vi "Compare Topologies.vi"(8 "error in (no error)":errorcluster, 9 "Modified Base Topology":path, 11 "Base Topology":path) -> (0 "error out":errorcluster, 3 "Differences":T2(array[cluster]) {"path capability" items=["Path Available"=1, "Path Exists"=2, "Path Unsupported"=3, "Resource in Use"=4, "Source Conflict"=5, "Channel Not Available"=6]; "path capability" items=["Path Available"=1, "Path Exists"=2, "Path Unsupported"=3, "Resource in Use"=4, "Source Conflict"=5, "Channel Not Available"=6]})   [LabVIEW 2017]
uses:
  <vilib>/SLSC_Switch/Path Capability.ctl
  <vilib>/SLSC_Switch/SLSC Switch.lvlib
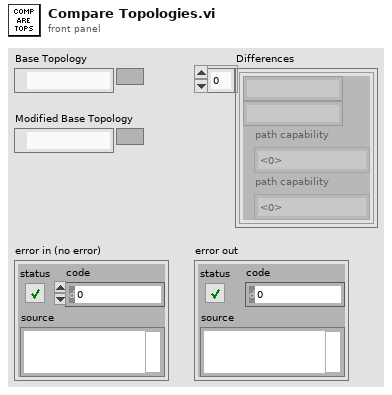
[diagram p1: front panel]
types:
  T1 = typedef "SLSC Switch.lvlib/Path Capability.ctl" = i32
  T2 = cluster{string, string, "path capability":T1, "path capability":T1}[]
  T3 = typedef "nislscslSession.ctl" = refnum<k20>
  T4 = cluster{string, string, "path capability":T1, "path capability":T1}
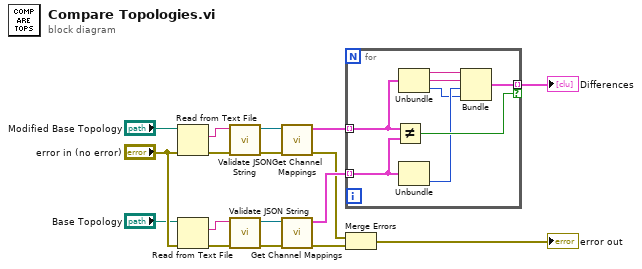
[diagram p0: block diagram]
diagram:
  n1 = Read from Text File(file (use dialog)="Modified Base Topology", error in="error in (no error)") -> (text=w2:string, error out=w6:errorcluster)  [unwired: 2 in, 2 out]
  n2 = Read from Text File(file (use dialog)="Base Topology", error in="error in (no error)") -> (text=w1:string, error out=w5:errorcluster)  [unwired: 2 in, 2 out]
  n3 = call "Validate JSON String.vi"("error in (no error)"=w6, "String"=w2) -> ("error out"=w13:errorcluster, "session out"=w12:T3)  [unwired: 8 in]
  n4 = call "Validate JSON String.vi"("error in (no error)"=w5, "String"=w1) -> ("error out"=w10:errorcluster, "session out"=w14:T3)  [unwired: 8 in]
  n5 = call "Get Channel Mappings.vi"("error in (no error)"=w13, "Refnum in"=w12) -> ("error out"=w9:errorcluster, "Channel Mappings"=w16:cluster{string, string, "path capability":T1}[])  [unwired: 8 in]
  n6 = call "Get Channel Mappings.vi"("error in (no error)"=w10, "Refnum in"=w14) -> ("error out"=w8:errorcluster, "Channel Mappings"=w15:cluster{string, string, "path capability":T1}[])  [unwired: 8 in]
  n7 = for {
    tunnel: w15 -> [w21] mode=indexing
    tunnel: w16 -> [w24] mode=indexing
    tunnel: [w20] -> w17 mode=indexing if=w25
    n8 = Not Equal?(x=w24, y=w21) -> (x != y?=w25:bool)
    n9 = Unbundle(w24) -> (w23:string, w22:string, "path capability"=w18:T1)
    n10 = Unbundle(w21) -> ("path capability"=w19:T1)  [unwired: 2 out]
    n11 = Bundle(w23, w22, "path capability"=w19, "path capability"=w18) -> (w20:T4)  [unwired: 1 in]
  }
  "Differences" <- w17
  n12 = Merge Errors(w9, w8) -> (→"error out":errorcluster)
